vi "xiLIB - SaveToINI_DIALOG.vi"(4 "Delay (ms)":u32=50, 6 "IniPath":path, 8 "error in (no error)":errorcluster, 9 "PRM[] to Save":T1[](array[typedef]), 11 "xiCam":refnum<k24>) -> (0 "error out":errorcluster, 3 "xiCam Out":refnum<k24>)   [LabVIEW 2013]
doc: "Dialog based parameter save function."
uses:
  xiCam/PRM/PRM/PRM_v2.ctl
  C:/Projects/Cameras3.x/xiLib/xiLIB_64bit/xiLIB/xiCamLib/API/x64/xiApi.NETX64.dll
  xiLIB_64bit/xiLIB/xiCamLib/API/x64/xiApi.NETX64.dll
  <vilib>/Utility/config.llb/Write Key (I32).vi
  <vilib>/Utility/config.llb/Write Key (Double).vi
  <vilib>/Utility/config.llb/Write Key (String).vi
  <vilib>/Utility/config.llb/NI_LVConfig.lvlib
panel:
  in  "STOP":bool
  in  "Slide":i32(slide) caption="Save Completed" min=0 scale=0.0..86.0
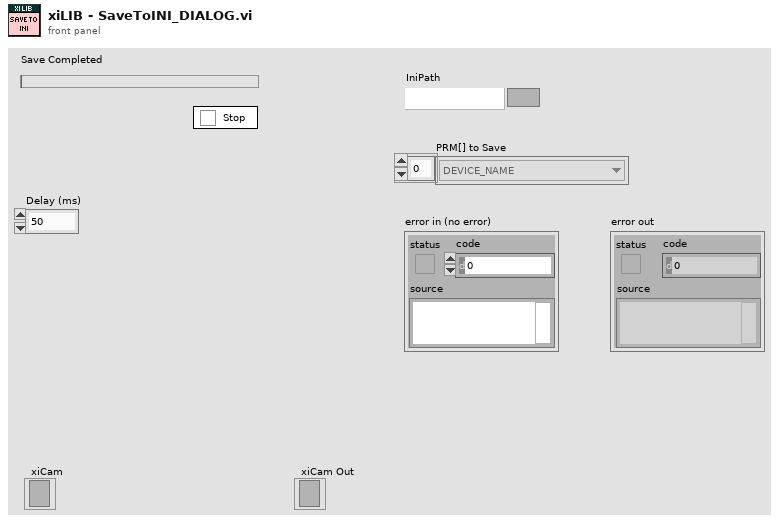
[diagram p1: front panel]
types:
  T1 = typedef "PRM_v2.ctl" = enum16{"ACQ_BUFFER_SIZE", "ACQ_FRAME_BURST_COUNT", "ACQ_TIMING_MODE", "ACQ_TRANSPORT_BUFFER_SIZE", "AE_MAX_LIMIT", "AEAG", "AEAG_LEVEL", "API_VERSION", "AG_MAX_LIMIT", "APPLY_CMS", "AUTO_BANDWIDTH_CALCULATION", "AUTO_WB", "AVAILABLE_BANDWIDTH", "AVAILABLE_BANDWIDTH_MAX", "AVAILABLE_BANDWIDTH_MIN", "BPC", "BUFFER_POLICY", "BUFFERS_QUEUE_SIZE", "CC_MATRIX_00", "CC_MATRIX_01", "CC_MATRIX_02", "CC_MATRIX_03", "CC_MATRIX_10", "CC_MATRIX_11", "CC_MATRIX_12", "CC_MATRIX_13", "CC_MATRIX_20", "CC_MATRIX_21", "CC_MATRIX_22", "CC_MATRIX_23", "CC_MATRIX_30", "CC_MATRIX_31", "CC_MATRIX_32", "CC_MATRIX_33", "CHIP_TEMP", "CMS", "COLOR_FILTER_ARRAY", "COOLING", "DEBOUNCE_EN", "DEBOUNCE_POL", "DEBOUNCE_T0", "DEBOUNCE_T1", "DEBUG_LEVEL", "DEFAULT_CC_MATRIX", "DEVICE_INSTANCE_PATH", "DEVICE_MODEL_ID", "DEVICE_NAME", "DEVICE_SN", "DEVICE_TYPE", "DEVICE_USER_ID", "DOWNSAMPLING", "DOWNSAMPLING_MAX", "DOWNSAMPLING_MIN", "DOWNSAMPLING_TYPE", "DRV_VERSION", "EXP_PRIORITY", "EXPOSURE", "EXPOSURE_DIRECT_UPDATE", "EXPOSURE_MAX", "EXPOSURE_MIN", "FFS_FILE_NAME", "FPGA1_VERSION", "FRAMERATE", "FRAMERATE_MAX", "FRAMERATE_MIN", "FREE_FFS_SIZE", "GAIN", "GAIN_DIRECT_UPDATE", "GAIN_MAX", "GAIN_MIN", "GAMMAC", "GAMMAY", "GPI_LEVEL", "GPI_MODE", "GPI_SELECTOR", "GPI_SELECTOR_MAX", "GPI_SELECTOR_MIN", "GPO_MODE", "GPO_SELECTOR", "GPO_SELECTOR_MAX", "GPO_SELECTOR_MIN", "HDR", "HDR_T1", "HDR_T2", "HEIGHT", "HEIGHT_MAX", "HEIGHT_MIN", "HOUSE_TEMP", "IMAGE_DATA_FORMAT", "IMAGE_IS_COLOR", "INPUT_CMS_PROFILE", "IS_COOLED", "IS_DEVICE_EXIST", "KNEEPOINT1", "KNEEPOINT2", "LED_MODE", "LED_SELECTOR", "LED_SELECTOR_MAX", "LED_SELECTOR_MIN", "LIMIT_BANDWIDTH", "LIMIT_BANDWIDTH_MAX", "LIMIT_BANDWIDTH_MIN", "LUT_EN", "LUT_INDEX", "LUT_INDEX_MAX", "LUT_INDEX_MIN", "LUT_VALUE", "LUT_VALUE_MAX", "LUT_VALUE_MIN", "MANUAL_WB", "MCU1_VERSION", "MCU2_VERSION", "OFFSET_X", "OFFSET_X_MAX", "OFFSET_X_MIN", "OFFSET_Y", "OFFSET_Y_MAX", "OFFSET_Y_MIN", "OUTPUT_CMS_PROFILE", "OUTPUT_DATA_BIT_DEPTH", "OUTPUT_DATA_PACKING", "READ_FILE_FFS", "RECENT_FRAME", "SENSOR_DATA_BIT_DEPTH", "SENSOR_MODE", "SENSOR_TAPS", "SHARPNESS", "SHUTTER_TYPE", "TARGET_TEMP", "TRG_DELAY", "TRG_SELECTOR", "TRG_SOFTWARE", "TRG_SOURCE", "USED_FFS_SIZE", "WB_KB", "WB_KG", "WB_KR", "WIDTH", "WIDTH_MAX", "WIDTH_MIN", "WRITE_FILE_FFS", "ACQ_BUFFER_SIZE_UNIT", "ACQ_TRANSPORT_BUFFER_COMMIT", "AEAG_ROI_HEIGHT", "AEAG_ROI_OFFSET_X", "AEAG_ROU_OFFSET_Y", "AEAG_ROI_WIDTH", "API_CONTEXT_LIST", "BINNING_HORIZONTAL", "BINNING_PATTERN", "BINNING_SELECTOR", "BINNING_VERTICAL", "COLUMN_FPN_CORRECTION", "COUNTER_SELECTOR", "COUNTER_VALUE", "DECIMATION_HORIZONTAL", "DECIMATION_PATTERN", "DECIMATION_SELECTOR", "DECIMATION_VERTICAL", "DEVICE_ID", "DEVICE_LOCATION_PATH", "DEVICE_MANIFEST", "DEVICE_RESET", "DEVICE_SENS_SN", "EXPOSURE_BURST_COUNT", "FFS_ACCESS_KEY", "GAIN_SELECTOR", "HW_REVISION", "IMAGE_BLACK_LEVEL", "IMAGE_DATA_BIT_DEPTH", "IMAGE_DATA_FORMAT_RGB32_ALPHA", "IMAGE_PAYLOAD_SIZE", "LENS_APERTURE_VALUE", "LENS_FEATURE", "LENS_FEATURE_SELECTOR", "LENS_FOCAL_LENGTH", "LENS_FOCUS_DISTANCE", "LENS_FOCUS_MOVE", "LENS_FOCUS_MOVEMENT_VALUE", "LENS_MODE", "OUTPUT_DATA_PACKING_TYPE", "SENSOR_CLOCK_FREQ_HZ", "SENSOR_CLOCK_FREQ_INDEX", "SENSOR_FEATURE_SELECTOR", "SENSOR_FEATURE_VALUE", "SENSOR_OUTPUT_CHANNEL_COUNT", "TRANSPORT_PIXEL_FORMAT", "TS_RST_MODE", "TS_RST_SOURCE"}
  T2 = typedef "NI_LVConfig.lvlib/Config Data RefNum.ctl" = refnum<k1>
  T3 = typedef "xiLIB - PRM_Attribute.ctl" = cluster{"Type":T4, "Method":T5, "Desc.":string, "PRM":T1}
  T4 = typedef "xiLIB - PRM_Type.ctl" = enum16{"Int32", "Float", "String", "DOWNSAMPLING_TYPE", "IMAGE_DATA_FORMAT", "BUFFER_POLICY", "TRG_SOURCE", "GPI", "GPO", "ACQ_TIMING_MODE", "BINNING_PATTERN", "BINNING_SELECTOR", "CMS_MODE", "COUNTER_SELECTOR", "DEBUG_LEVEL", "DECIMATION_PATTERN", "DECIMATION_SELECTOR", "GAIN_SELECTOR_TYPE", "LED_MODE", "LENS_FEATURE_SELECTOR", "LENS_MODE", "OUTPUT_DATA_PACKING_TYPE", "SENSOR_FEATURE_SELECTOR", "SHUTTER_TYPE", "TRG_SELECTOR", "TS_RST_MODE", "TS_RST_SOURCE"}
  T5 = typedef "xiLIB - PRM_Function.ctl" = enum16{"Get / Set", "Get", "Set"}
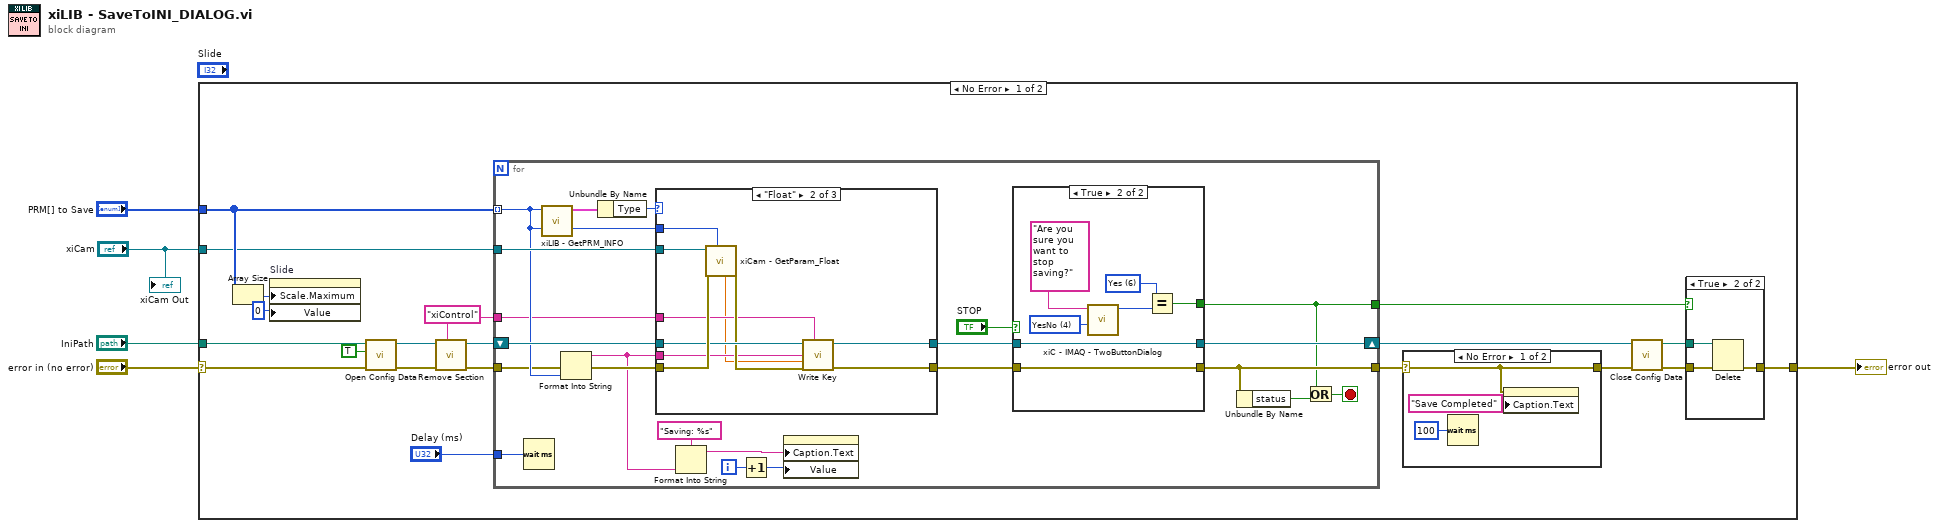
[diagram p0: block diagram]
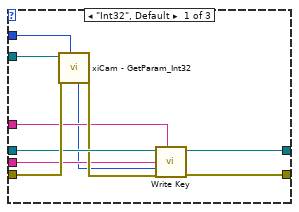
[diagram p5: hidden frame]
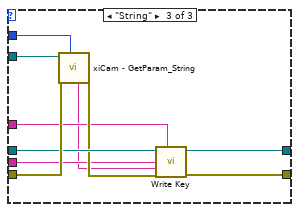
[diagram p6: hidden frame]
diagram:
  n1 = case shown="No Error" "error in (no error)" {
    selector: "error in (no error)" -> [w24 w95]
    tunnel: [w11 w95] -> w4
    tunnel: "IniPath" -> [w25 _]
    tunnel: "PRM[] to Save" -> [w16 _]
    tunnel: "xiCam" -> [w9 _]
    frame No Error {
      w18 = "xiControl" ("section")
      n2 = Array Size(array=w16) -> (size(s)=w15:i32)
      n3 = property on="Slide" class="Slide (strict)"("Scale.Maximum"=w15, "Value"=0 ("Slide")) -> ()  [unwired: 2 in, 2 out]
      n4 = call <vilib>:"Open Config Data.vi"("error in (no error)"=w24, "create file if necessary (T)"=TRUE, "configuration file path"=w25) -> ("error out"=w22:errorcluster, "refnum"=w21:T2)  [unwired: 6 in, 1 out]
      n5 = call <vilib>:"Remove Section.vi"("section"=w18, "error in (no error)"=w22, "refnum"=w21) -> ("error out"=w19:errorcluster, "refnum out"=w20:T2)  [unwired: 6 in, 1 out]
      n6 = for {
        tunnel: w9 -> [w53]
        tunnel: w16 -> [w51] mode=indexing
        tunnel: w19 -> [w50]
        tunnel: w18 -> [w48]
        shift-right: [w39] -> w17
        shift-left: w20 -> [w52]
        tunnel: [w37] -> w7
        tunnel: [w35] -> w14
        tunnel: "Delay (ms)" -> [w34]
        i -> [w47]
        stop <- w36 stop-if-true
        n7 = Wait (ms)(milliseconds to wait=w34) -> ()  [unwired: 1 out]
        n8 = call "xiLIB - GetPRM_INFO.vi"("PRM"=w51) -> ("PRM_Attributes"=w55:T3)  [unwired: 10 in]
        n9 = Format Into String(error in=w50, w51) -> (resulting string=w44:string, error out=w49:errorcluster)  [unwired: 2 in]
        n10 = Unbundle By Name(w55) -> ("Type"=w54:T4)
        n11 = case shown="\"Float\"" w54 {
          tunnel: w53 -> [w65 w75 w85]
          tunnel: w51 -> [w74 w84 w94]
          tunnel: w49 -> [w73 w83 w93]
          tunnel: w52 -> [w72 w82 w92]
          tunnel: w44 -> [w70 w80 w90]
          tunnel: w48 -> [w69 w79 w89]
          tunnel: [w67 w77 w87] -> w42
          tunnel: [w66 w76 w86] -> w41
          frame "Int32", Default {
            n12 = call "xiCam - GetParam_Int32.vi"("PRM"=w74, "error in (no error)"=w73, "xiCam In"=w65) -> ("error out"=w71:errorcluster, "Int32_Value"=w68:i32)  [unwired: 6 in, 1 out]
            n13 = call-poly <vilib>:"Write Key.vi"("section"=w69, "error in (no error)"=w71, "value"=w68, "key"=w70, "refnum"=w72) -> ("error out"=w66:errorcluster, "refnum out"=w67:T2)  [unwired: 4 in, 1 out]
          }
          frame "Float" {
            n14 = call "xiCam - GetParam_Float.vi"("PRM"=w84, "error in (no error)"=w83, "xiCam In"=w75) -> ("error out"=w81:errorcluster, "Float_Value"=w78:sgl)  [unwired: 6 in, 1 out]
            n15 = call-poly <vilib>:"Write Key.vi"("section"=w79, "error in (no error)"=w81, "value"=w78, "key"=w80, "refnum"=w82) -> ("error out"=w76:errorcluster, "refnum out"=w77:T2)  [unwired: 4 in, 1 out]
          }
          frame "String" {
            n16 = call "xiCam - GetParam_String.vi"("PRM"=w94, "error in (no error)"=w93, "xiCam In"=w85) -> ("error out"=w91:errorcluster, "String_Value"=w88:string)  [unwired: 6 in, 1 out]
            n17 = call-poly <vilib>:"Write Key.vi"("section"=w89, "error in (no error)"=w91, "value"=w88, "key"=w90, "refnum"=w92) -> ("error out"=w86:errorcluster, "refnum out"=w87:T2)  [unwired: 4 in, 1 out]
          }
        }
        n18 = Format Into String(format string="Saving: %s", w44) -> (resulting string=w43:string)  [unwired: 2 in, 1 out]
        n19 = Increment(x=w47) -> (x+1=w46:i32)
        n20 = property on="Slide" class="Slide (strict)"("Caption.Text"=w43, "Value"=w46) -> ()  [unwired: 2 in, 2 out]
        n21 = case shown="True" "STOP" {
          tunnel: w42 -> [w57 w62]
          tunnel: w41 -> [w56 w61]
          tunnel: [w57 w62] -> w39
          tunnel: [w56 w61] -> w37
          tunnel: [_ w58] -> w35
          frame False {
          }
          frame True {
            w59 = 6 items=["None", "OK", "Cancel", "Abort", "Retry", "Ignore", "Yes", "No"] ("Show")
            w63 = 4 items=["OK", "OKCancel", "AbortRetryIgnore", "YesNoCancel", "YesNo", "RetryCancel"] ("Button")
            n22 = call "xiC - IMAQ - TwoButtonDialog.vi"("Button"=w63, "Text"="Are you sure you want to stop saving?") -> ("Show"=w60:i32)  [unwired: 8 in, 1 out]
            n23 = Equal?(x=w59, y=w60) -> (x = y?=w58:bool)
          }
        }
        n24 = Unbundle By Name(w37) -> ("status"=w38:bool)
        n25 = Or(x=w35, y=w38) -> (x .or. y?=w36:bool)
      }
      n26 = case shown="No Error" w7 {
        selector: w7 -> [w27 w29]
        tunnel: [w27 w29] -> w6
        frame No Error {
          n27 = Wait (ms)(milliseconds to wait=u32 100) -> ()  [unwired: 1 out]
          n28 = property on="Slide" class="Slide (strict)"(error in=w27, "Caption.Text"="Save Completed") -> ()  [unwired: 1 in, 2 out]
        }
        frame Error {
        }
      }
      n29 = call <vilib>:"Close Config Data.vi"("error in (no error)"=w6, "refnum"=w17) -> ("error out"=w12:errorcluster, "file path"=w13:path)  [unwired: 8 in]
      n30 = case shown="True" w14 {
        tunnel: w13 -> [_ w33]
        tunnel: w12 -> [w30 w32]
        tunnel: [w30 w31] -> w11
        frame False {
        }
        frame True {
          n31 = Delete(path (use dialog)=w33, error in=w32) -> (error out=w31:errorcluster)  [unwired: 3 in, 2 out]
        }
      }
    }
    frame Error {
    }
  }
  "error out" <- w4
  "xiCam Out" <- "xiCam"
